vi "Interface.vi"(0 "Data In":T4 {"time" format="%<%H:%M:%S%2u>T"}, 2 "Display State In":T2, 3 "Container State":T3) -> (6 "Data Out":T4 {"time" format="%<%H:%M:%S%2u>T"}, 7 "Display State Out":T2, 8 "Action":T1)   [LabVIEW 2016, in "1D Buffer.xctl"]
uses:
  1D Buffer.xctl
  Data.ctl
  <vilib>/_xctls/Container State.ctl
  State.ctl
  <vilib>/_xctls/Action.ctl
  <vilib>/_xctls/XControlSupport.lvlib
panel:
  out "Data":cluster{"Time Array":timestamp[], sgl[]}(graph)
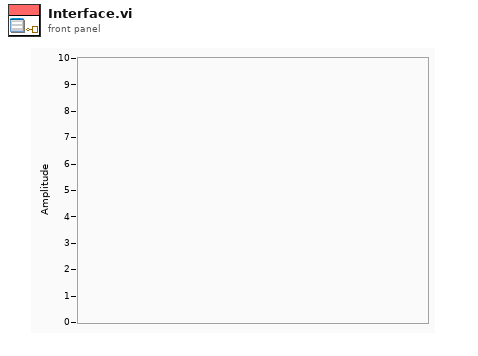
[diagram p1: front panel]
types:
  T1 = typedef "XControlSupport.lvlib/Action.ctl" = cluster{"Data Changed?":bool, "State Changed?":bool, "Action Name":string}
  T2 = typedef "1D Buffer.xctl/State.ctl" = cluster{"Data Array":sgl[][], "Time Array":timestamp[], "History":u16, "Variable":bool[], "Plot Details":cluster{"Name":string, "Line Width":u8, "Line Style":u8, "Color":u32}[], "Y-Axis Labels":string[], "legend visible":bool}
  T3 = typedef "XControlSupport.lvlib/Container State.ctl" = cluster{"Indicator?":bool, "Run Mode?":bool, " Refnum":refnum<vi>}
  T4 = typedef "1D Buffer.xctl/Data.ctl" = cluster{"time":timestamp, "data":sgl[]}
  T5 = cluster{"Name":string, "Line Width":u8, "Line Style":u8, "Color":u32}[]
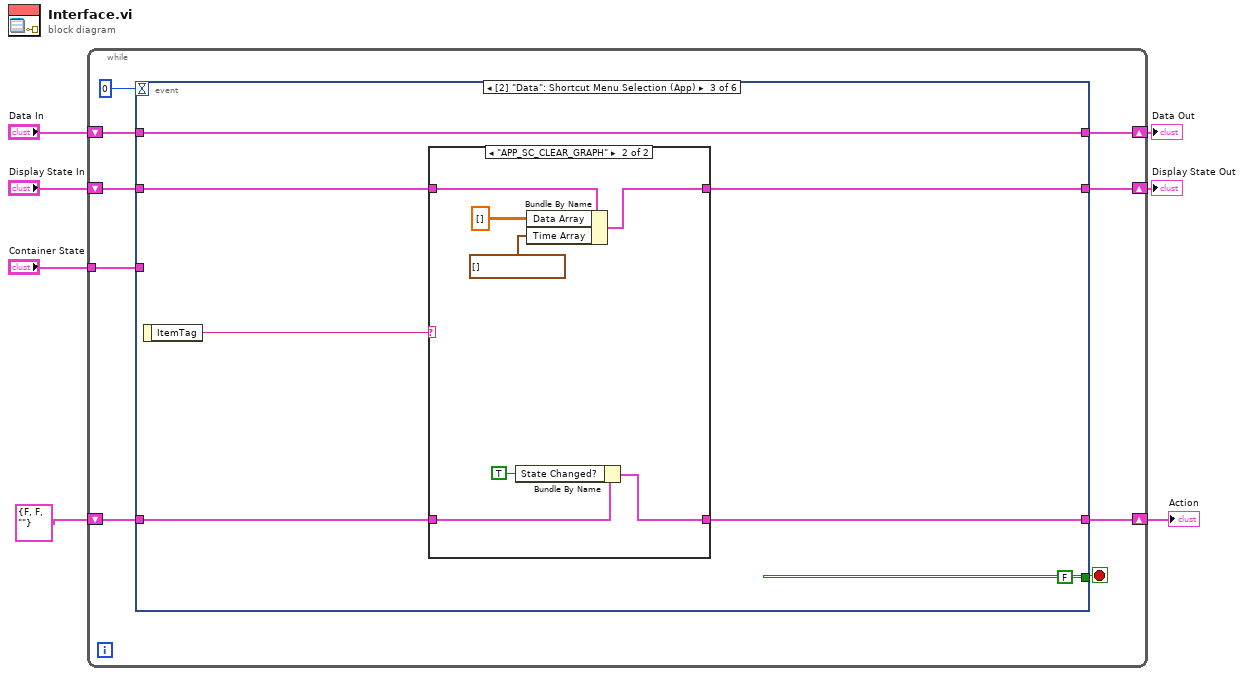
[diagram p0: block diagram]
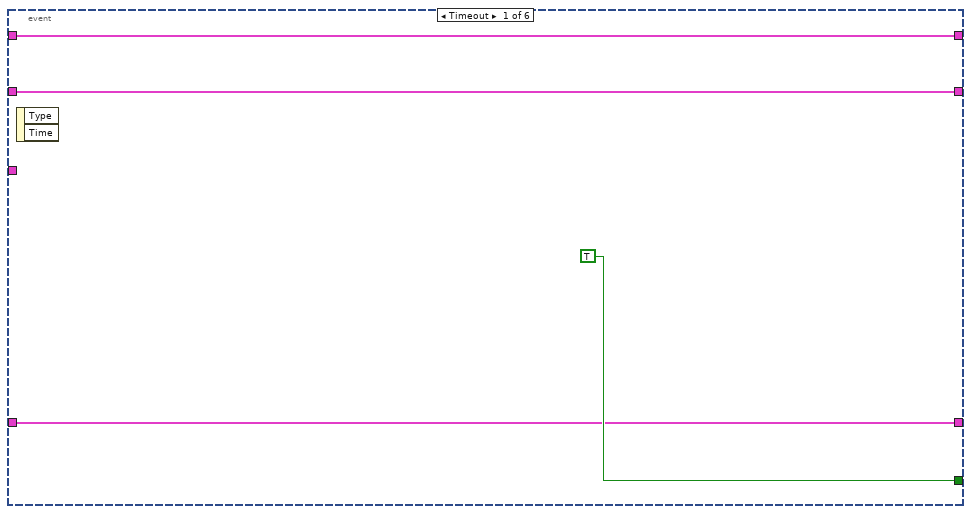
[diagram p2: hidden frame]
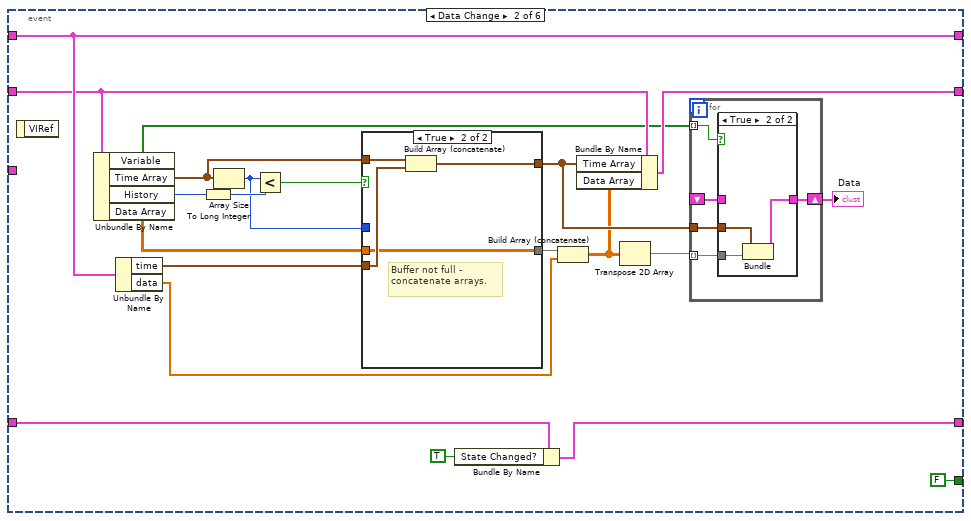
[diagram p3: hidden frame]
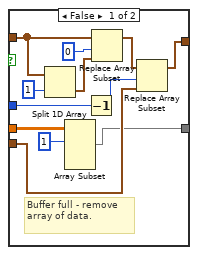
[diagram p5: hidden frame]
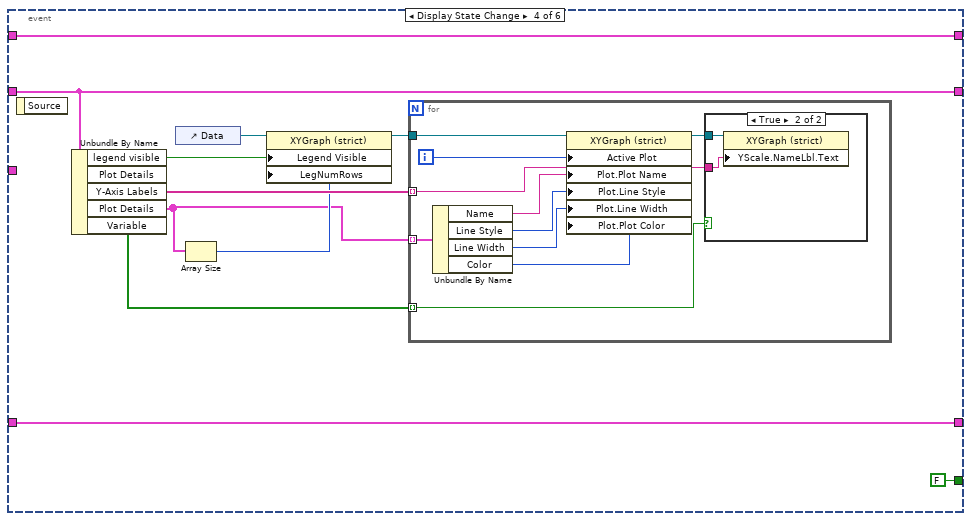
[diagram p7: hidden frame]
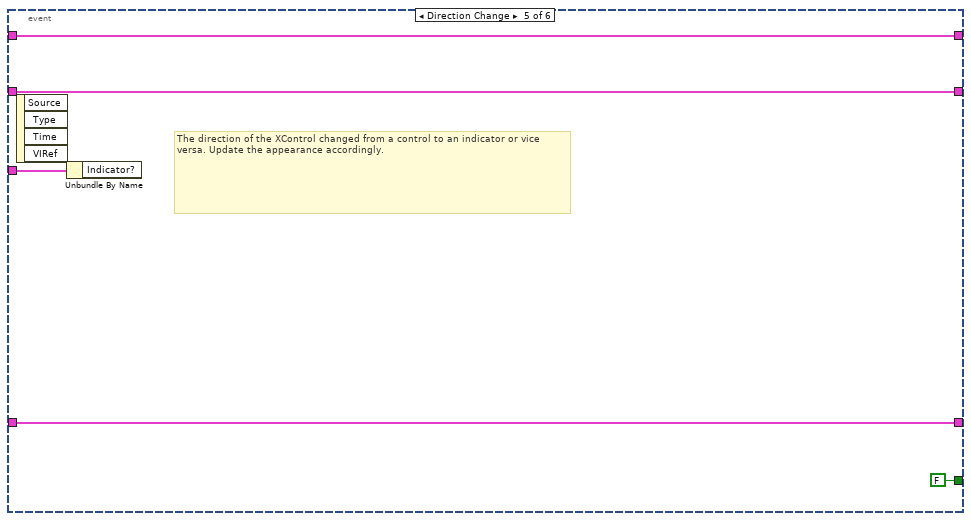
[diagram p9: hidden frame]
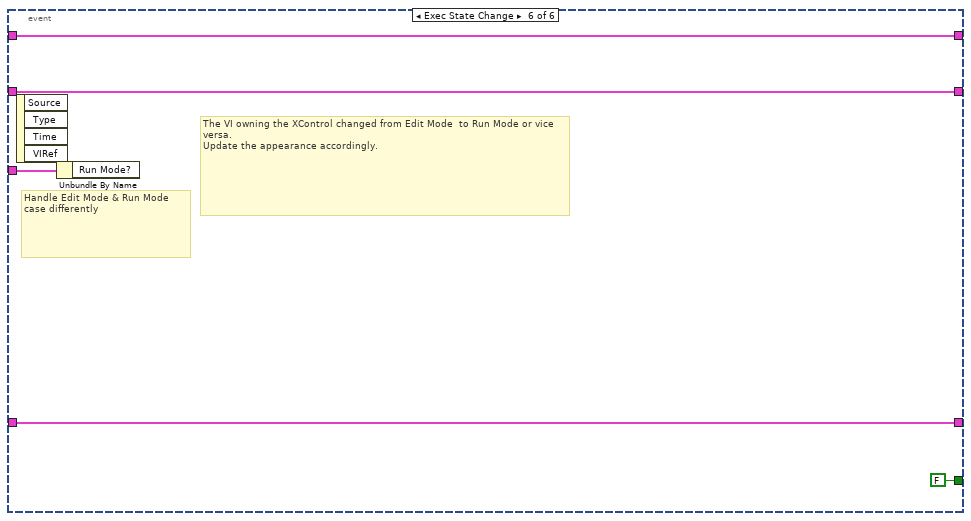
[diagram p10: hidden frame]
diagram:
  n1 = while {
    shift-right: [w15] -> w4
    shift-left: "Display State In" -> [w16]
    tunnel: "Container State" -> [w12]
    shift-right: [w10] -> w7
    shift-left: "Data In" -> [w11]
    shift-right: [w8] -> w2
    shift-left: T1 {"Data Changed?"=FALSE, "State Changed?"=FALSE, "Action Name"=""} ("Action") -> [w9]
    stop <- w14 stop-if-true
    n2 = event shown="[2] \"Data\": Shortcut Menu Selection (App)" {
      selector: _ -> [_ _ _ _ _ _]
      dyn-events: _ -> [_ _ _ _ _ _]
      timeout: 0 -> [_ _ _ _ _ _]
      tunnel: w16 -> [w18 w33 w71 w91 w109 w114]
      tunnel: [w18 w32 w70 w91 w109 w114] -> w15
      tunnel: [TRUE FALSE FALSE FALSE FALSE FALSE] -> w14
      tunnel: w12 -> [_ _ _ _ w110 w115]
      tunnel: w11 -> [w17 w41 w73 w93 w108 w113]
      tunnel: [w17 w41 w73 w93 w108 w113] -> w10
      tunnel: [w19 w27 w68 w92 w107 w112] -> w8
      tunnel: w9 -> [w19 w29 w69 w92 w107 w112]
      event Timeout {
        n3 = event-data() -> ()  [unwired: 1 in, 2 out]
      }
      event Data Change {
        n4 = event-data() -> ()  [unwired: 1 in, 1 out]
        n5 = Unbundle By Name(w33) -> ("Variable"=w26:bool[], "Time Array"=w38:timestamp[], "History"=w40:u16, "Data Array"=w36:sgl[][])
        n6 = Unbundle By Name(w41) -> ("time"=w37:timestamp, "data"=w24:sgl[])
        n7 = To Long Integer(number=w40) -> (32bit integer=w35:i32)
        n8 = Array Size(array=w38) -> (size(s)=w34:i32)
        n9 = Less?(x=w34, y=w35) -> (x < y?=w39:bool)
        n10 = case shown="True" w39 {
          tunnel: w38 -> [w57 w66]
          tunnel: [w56 w64] -> w31
          tunnel: w37 -> [w55 w65]
          tunnel: w36 -> [w52 w63]
          tunnel: w34 -> [w54 _]
          tunnel: [w51 w63] -> w25
          frame False {
            # "Buffer full - remove array of data."
            n11 = Split 1D Array(array=w57, index=1) -> (second subarray=w58:timestamp[])  [unwired: 1 out]
            n12 = Array Subset(array=w52, index (row)=1 ("index")) -> (w51:sgl[][])  [unwired: 3 in]
            n13 = Decrement(x=w54) -> (x-1=w60:i32)
            n14 = Replace Array Subset(array=w57, new element=w58, index=0) -> (w61:timestamp[])
            n15 = Replace Array Subset(array=w61, new element=w55, index=w60) -> (w56:timestamp[])
          }
          frame True {
            # "Buffer not full - concatenate arrays."
            n16 = Build Array (concatenate)(w66, w65) -> (w64:timestamp[])
          }
        }
        n17 = Bundle By Name(cluster=w29, "State Changed?"=TRUE) -> (w27:T1)
        n18 = Build Array (concatenate)(w25, w24) -> (w22:sgl[][])
        n19 = Bundle By Name(cluster=w33, "Time Array"=w31, "Data Array"=w22) -> (w32:T2)
        n20 = Transpose 2D Array(2D array=w22) -> (transposed array=w23:sgl[][])
        n21 = for {
          tunnel: w31 -> [w46]
          tunnel: w23 -> [w44] mode=indexing
          tunnel: w26 -> [w43] mode=indexing
          shift-right: [w45] -> w30
          shift-left: _ -> [w42]
          n22 = case shown="True" w43 {
            tunnel: w46 -> [_ w50]
            tunnel: [w47 w49] -> w45
            tunnel: w44 -> [_ w48]
            tunnel: w42 -> [w47 _]
            frame False {
            }
            frame True {
              n23 = Bundle("Time Array"=w50, w48) -> (w49:cluster{"Time Array":timestamp[], sgl[]})  [unwired: 1 in]
            }
          }
        }
        "Data" <- w30
      }
      event "Data": Shortcut Menu Selection (App) {
        n24 = event-data() -> ("ItemTag"=w72:string)  [unwired: 1 in]
        n25 = case shown="\"APP_SC_CLEAR_GRAPH\"" w72 {
          tunnel: w71 -> [w75 w82]
          tunnel: [w75 w79] -> w70
          tunnel: w69 -> [w74 w78]
          tunnel: [w74 w76] -> w68
          frame "False", Default {
          }
          frame "APP_SC_CLEAR_GRAPH" {
            n26 = Bundle By Name(cluster=w78, "State Changed?"=TRUE) -> (w76:T1)
            n27 = Bundle By Name(cluster=w82, "Data Array"=sgl[][] [], "Time Array"=timestamp[] []) -> (w79:T2)
          }
        }
      }
      event Display State Change {
        n28 = event-data() -> ()  [unwired: 1 in, 1 out]
        n29 = Unbundle By Name(w91) -> ("legend visible"=w90:bool, "Y-Axis Labels"=w87:string[], "Plot Details"=w84:T5, "Variable"=w85:bool[])  [unwired: 1 out]
        n30 = control-ref of="Data"() -> (w89:refnum<vi>)
        n31 = Array Size(array=w84) -> (size(s)=w86:i32)
        n32 = property on="Property Node" class="XYGraph (strict)"(reference=w89, "Legend Visible"=w90, "LegNumRows"=w86) -> (reference out=w88:refnum<vi>)  [unwired: 1 in, 1 out]
        n33 = for {
          tunnel: w88 -> [w103]
          tunnel: w84 -> [w101] mode=indexing
          tunnel: w85 -> [w95] mode=indexing
          tunnel: w87 -> [w94] mode=indexing
          i -> [w102]
          n34 = Unbundle By Name(w101) -> ("Name"=w100:string, "Line Style"=w99:u8, "Line Width"=w98:u8, "Color"=w97:u32)
          n35 = property on="Property Node" class="XYGraph (strict)"(reference=w103, "Active Plot"=w102, "Plot.Plot Name"=w100, "Plot.Line Style"=w99, "Plot.Line Width"=w98, "Plot.Plot Color"=w97) -> (reference out=w96:refnum<vi>)  [unwired: 1 in, 1 out]
          n36 = case shown="True" w95 {
            tunnel: w96 -> [_ w104]
            tunnel: w94 -> [_ w105]
            frame False {
            }
            frame True {
              n37 = property on="Property Node" class="XYGraph (strict)"(reference=w104, "YScale.NameLbl.Text"=w105) -> ()  [unwired: 1 in, 2 out]
            }
          }
        }
      }
      event Direction Change {
        # "The direction of the XControl changed from a control to an indicator or vice versa. Update the appearance accordingly."
        n38 = event-data() -> ()  [unwired: 1 in, 4 out]
        n39 = Unbundle By Name(w110) -> ()  [unwired: 1 out]
      }
      event Exec State Change {
        # "The VI owning the XControl changed from Edit Mode  to Run Mode or vice versa.\nUpdate the appearance accordingly."
        # "Handle Edit Mode & Run Mode\ncase differently"
        n40 = event-data() -> ()  [unwired: 1 in, 4 out]
        n41 = Unbundle By Name(w115) -> ()  [unwired: 1 out]
      }
    }
  }
  "Display State Out" <- w4
  "Data Out" <- w7
  "Action" <- w2
